vi "CRYRub & Buzz total Loudness.vi"(6 "number":i32, 8 "Fsp[k]":dbl[](array[numeric]), 9 "size":i32, 10 "Version":i32, 11 "Real matrix":dbl[][](array[numeric])) -> (4 "E2[k]":dbl[](array[numeric]))   [LabVIEW 2013]
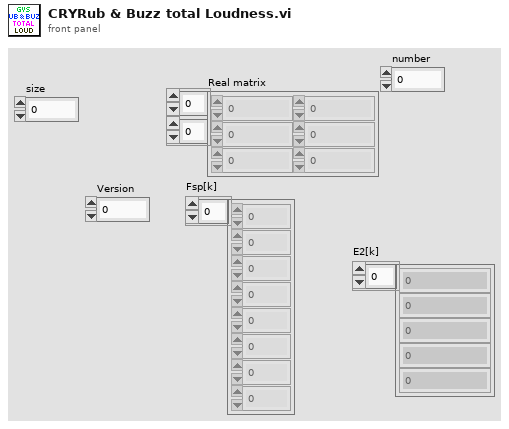
[diagram p1: front panel]
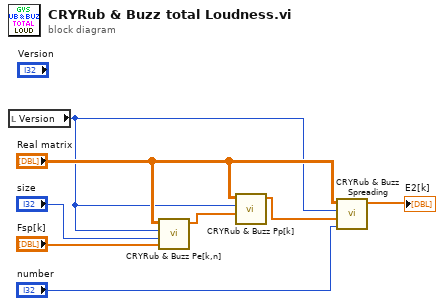
[diagram p0: block diagram]
diagram:
  n1 = local read "Version"() -> (w6:i32)
  n2 = call "CRYRub & Buzz Pe[k,n].vi"("Real matrix"="Real matrix", "Version"=w6, "size"="size", "Fsp[k]"="Fsp[k]") -> ("Pe[k]"=w2:dbl[])  [unwired: 4 in]
  n3 = call "CRYRub & Buzz Pp[k].vi"("Pe[k]"=w2, "Version"=w6, "Real matrix"="Real matrix") -> ("Pp[k]"=w1:dbl[])  [unwired: 7 in]
  n4 = call "CRYRub & Buzz Spreading.vi"("number"="number", "Pp[k]"=w1, "Version"=w6, "Real matrix"="Real matrix") -> ("E2[k]"=→"E2[k]":dbl[])  [unwired: 7 in]
